vi "wait_03.vi"() -> (1 "Wait time remaining (s)":string, 2 "Done":bool)   [LabVIEW 2011]
uses:
  wait_globals.vi
panel:
  out "Total wait time (s)":string
  out "wait time remaining (s)":dbl
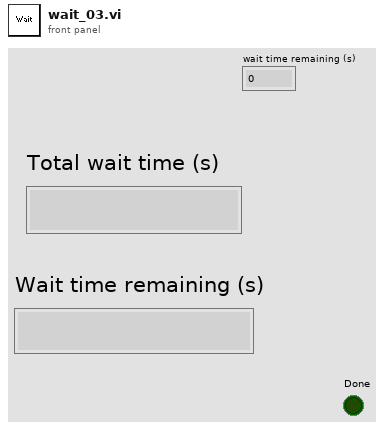
[diagram p1: front panel]
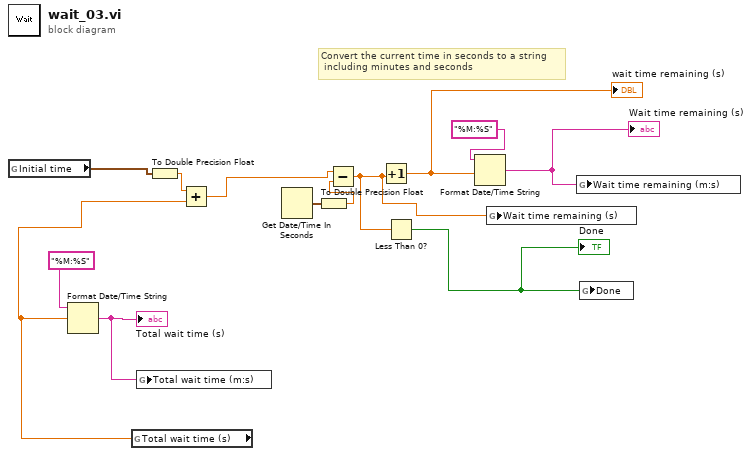
[diagram p0: block diagram]
diagram:
  # "Convert the current time in seconds to a string\n including minutes and seconds"
  n1 = global read "wait_globals.vi" "Initial time"() -> (w1:timestamp)
  n2 = global read "wait_globals.vi" "Total wait time (s)"() -> (w10:dbl)
  n3 = Format Date/Time String(time format string (%c)="%M:%S", seconds (now)=w10) -> (date/time string=w11:string)  [unwired: 1 out]
  "Total wait time (s)" <- w11
  n4 = global write "wait_globals.vi" "Total wait time (m:s)"(w11) -> ()
  n5 = To Double Precision Float(number=w1) -> (double precision float=w13:dbl)
  n6 = Add(x=w13, y=w10) -> (x+y=w2:dbl)
  n7 = Get Date/Time In Seconds() -> (seconds since 1Jan1904=w5:timestamp)
  n8 = To Double Precision Float(number=w5) -> (double precision float=w4:dbl)
  n9 = Subtract(x=w2, y=w4) -> (x-y=w8:dbl)
  n10 = Increment(x=w8) -> (x+1=w7:dbl)
  "wait time remaining (s)" <- w7
  n11 = Less Than 0?(x=w8) -> (x < 0?=w6:bool)
  "Done" <- w6
  n12 = Format Date/Time String(time format string (%c)="%M:%S", seconds (now)=w7) -> (date/time string=w9:string)  [unwired: 1 out]
  "Wait time remaining (s)" <- w9
  n13 = global write "wait_globals.vi" "Wait time remaining (s)"(w8) -> ()
  n14 = global write "wait_globals.vi" "Wait time remaining (m:s)"(w9) -> ()
  n15 = global write "wait_globals.vi" "Done"(w6) -> ()
